vi "showItems.vi"(8 "error in (no error)":errorcluster, 11 "Meal in":refnum<class "Meal.lvclass">) -> (0 "error out":errorcluster, 3 "Meal out":refnum<class "Meal.lvclass">)   [LabVIEW 2017, in "Meal.lvclass"]
uses:
  Meal.lvclass
  ConsoleOut/Print Options.ctl
  Meal.lvclass/Meal.ctl
  Item Class/Item.lvclass
  Packing Class/Packing.lvclass
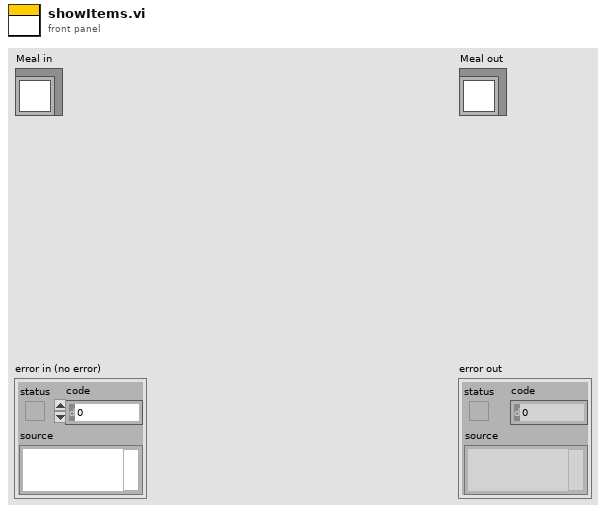
[diagram p1: front panel]
types:
  T1 = typedef "Print Options.ctl" = enum16{"Create", "Get Reference", "Print", "Print Header", "Close"}
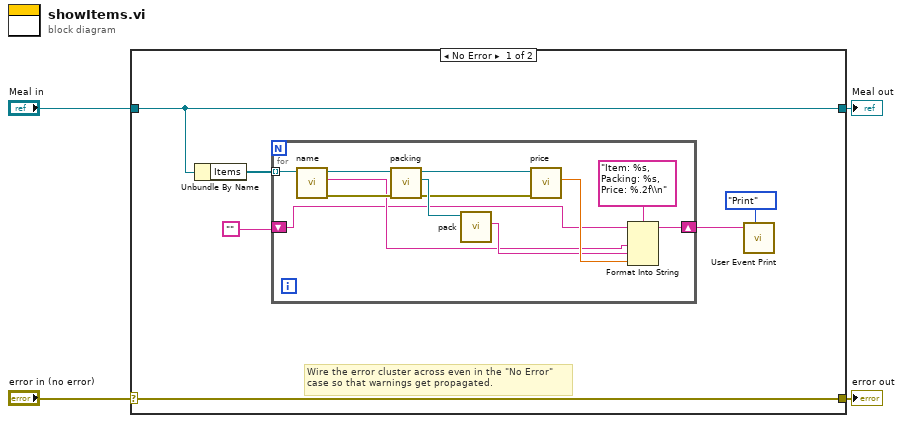
[diagram p0: block diagram]
diagram:
  n1 = case shown="No Error" "error in (no error)" {
    selector: "error in (no error)" -> [w10 w24]
    tunnel: [w10 w24] -> w3
    tunnel: [w9 w23] -> w1
    tunnel: "Meal in" -> [w9 w23]
    frame No Error {
      # "Wire the error cluster across even in the \"No Error\"\ncase so that warnings get propagated."
      n2 = Unbundle By Name(w9) -> ("Items"=w8:refnum<class "Item.lvclass">[])
      n3 = for {
        tunnel: w8 -> [w22] mode=indexing
        shift-right: [w11] -> w6
        shift-left: "" -> [w12]
        n4 = call-dynamic "name.vi"("Item in"=w22) -> ("error out"=w21:errorcluster, "name"=w13:string, "Item out"=w20:refnum<class "Item.lvclass">)  [unwired: 8 in]
        n5 = call-dynamic "packing.vi"("error in (no error)"=w21, "Item in"=w20) -> ("error out"=w17:errorcluster, "Packing.lvclass"=w19:refnum<class "Packing.lvclass">, "Item out"=w18:refnum<class "Item.lvclass">)  [unwired: 7 in]
        n6 = call-dynamic "pack.vi"("Packing in"=w19) -> ("Packing"=w14:string)  [unwired: 8 in, 2 out]
        n7 = call-dynamic "price.vi"("error in (no error)"=w17, "Item in"=w18) -> ("price"=w15:dbl)  [unwired: 7 in, 2 out]
        n8 = Format Into String(format string="Item: %s, Packing: %s, Price: %.2f\\n", initial string=w12, w13, w14, w15) -> (resulting string=w11:string)  [unwired: 1 in, 1 out]
      }
      n9 = call "User Event Print.vi"("Options"=Print_Options."Print", "String to Print"=w6) -> ()  [unwired: 8 in, 2 out]
    }
    frame Error {
    }
  }
  "error out" <- w3
  "Meal out" <- w1
